vi "DPD Measure.vi"(0 "RFmx Handle In":refnum<k21>, 1 "Selector String":string, 5 "Previous DPD Polynomial":csg[](array[numeric]), 11 "error in (no error)":errorcluster) -> (4 "RFmx Handle Out":refnum<k21>, 6 "DPD Results":T1 {"DPD Polynomial" format="%.2f"; "NMSE (dB)" format="%.2f"; "Average Gain (dB)" format="%.2f"}, 8 "Selector String Out":string, 15 "error out":errorcluster)   [LabVIEW 2016, in "RFmxSpecAn.lvlib"]
uses:
  RFmxSpecAn.lvlib
  Typedefs/DPD Results.ctl
  <vilib>/RFmx/SpecAn/mx/RFmxSpecAn.llb/RFmxSpecAn Select Measurement (Single).vi
  <vilib>/RFmx/SpecAn/mx/RFmxSpecAn.llb/RFmxSpecAn DPD Fetch DPD Polynomial.vi
  <vilib>/RFmx/SpecAn/mx/RFmxSpecAn.llb/RFmxSpecAn DPD Fetch Lookup Table.vi
  <vilib>/RFmx/SpecAn/mx/RFmxSpecAn.llb/RFmxSpecAn DPD Fetch NMSE.vi
  <vilib>/RFmx/SpecAn/mx/RFmxSpecAn.llb/RFmxSpecAn DPD Fetch Average Gain.vi
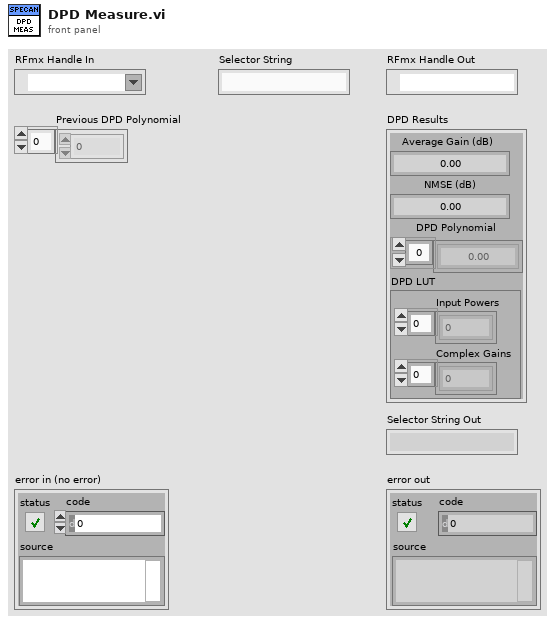
[diagram p1: front panel]
types:
  T1 = typedef "RFmxSpecAn.lvlib/DPD Results.ctl" = cluster{"Average Gain (dB)":dbl, "NMSE (dB)":dbl, "DPD Polynomial":csg[], "DPD LUT":cluster{"Input Powers":sgl[], "Complex Gains":csg[]}}
  T2 = enum16{"ACP", "CCDF", "CHP", "FCnt", "Harmonics", "OBW", "SEM", "Spectrum", "Spur", "TXP", "AMPM", "DPD", "IQ", "IM", "NF", "PhaseNoise"}
  T3 = cluster{"Input Powers":sgl[], "Complex Gains":csg[]}
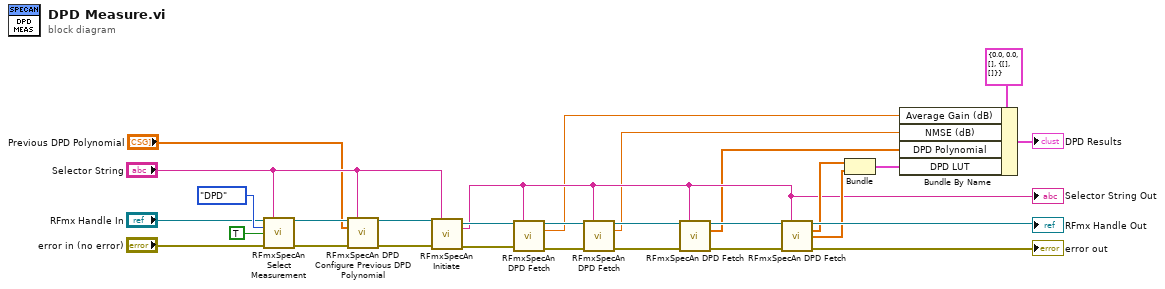
[diagram p0: block diagram]
diagram:
  n1 = call-poly <vilib>:"RFmxSpecAn Select Measurement.vi"("Instrument Handle In"="RFmx Handle In", "Selector String"="Selector String", "Measurement"=T2."DPD", "Enable All Traces"=TRUE, "error in (no error)"="error in (no error)") -> ("Instrument Handle Out"=w4:refnum<k21>, "error out"=w25:errorcluster)  [unwired: 9 in]
  n2 = call <vilib>:"RFmxSpecAn DPD Configure Previous DPD Polynomial.vi"("Instrument Handle In"=w4, "Selector String"="Selector String", "Previous DPD Polynomial"="Previous DPD Polynomial", "error in (no error)"=w25) -> ("Instrument Handle Out"=w3:refnum<k21>, "error out"=w5:errorcluster)  [unwired: 10 in]
  n3 = call <vilib>:"RFmxSpecAn Initiate.vi"("Instrument Handle In"=w3, "Selector String"="Selector String", "error in (no error)"=w5) -> ("Instrument Handle Out"=w23:refnum<k21>, "Selector String Out"=w11:string, "error out"=w24:errorcluster)  [unwired: 10 in]
  "Selector String Out" <- w11
  n4 = call-poly <vilib>:"RFmxSpecAn DPD Fetch.vi"("Instrument Handle In"=w23, "Selector String"=w11, "error in (no error)"=w24) -> ("Instrument Handle Out"=w20:refnum<k21>, "Average Gain (dB)"=w6:dbl, "error out"=w22:errorcluster)  [unwired: 10 in]
  n5 = call-poly <vilib>:"RFmxSpecAn DPD Fetch.vi"("Instrument Handle In"=w20, "Selector String"=w11, "error in (no error)"=w22) -> ("Instrument Handle Out"=w18:refnum<k21>, "NMSE (dB)"=w7:dbl, "error out"=w21:errorcluster)  [unwired: 10 in]
  n6 = call-poly <vilib>:"RFmxSpecAn DPD Fetch.vi"("Instrument Handle In"=w18, "Selector String"=w11, "error in (no error)"=w21) -> ("Instrument Handle Out"=w16:refnum<k21>, "DPD Polynomial"=w8:csg[], "error out"=w19:errorcluster)  [unwired: 10 in]
  n7 = call-poly <vilib>:"RFmxSpecAn DPD Fetch.vi"("Instrument Handle In"=w16, "Selector String"=w11, "error in (no error)"=w19) -> ("Instrument Handle Out"=→"RFmx Handle Out":refnum<k21>, "Input Powers"=w14:sgl[], "Complex Gains"=w13:csg[], "error out"=→"error out":errorcluster)  [unwired: 9 in]
  n8 = Bundle("Input Powers"=w14, "Complex Gains"=w13) -> (w10:T3)  [unwired: 1 in]
  n9 = Bundle By Name(cluster=T1 {"Average Gain (dB)"=0.0, "NMSE (dB)"=0.0, "DPD Polynomial"=[], "DPD LUT"={"Input Powers"=[], "Complex Gains"=[]}} ("DPD Results"), "Average Gain (dB)"=w6, "NMSE (dB)"=w7, "DPD Polynomial"=w8, "DPD LUT"=w10) -> (→"DPD Results":T1)
